vi "AMI Request Compose.vi"(7 "Checksum used":bool=TRUE, 11 "Address":u8=1) -> (3 "Request":string, 4 "Command":string="AMI")   [LabVIEW 2015, in "Samwontech TEMP2xxx.lvlib"]
uses:
  Samwontech TEMP2xxx.lvlib
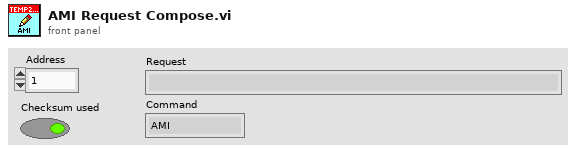
[diagram p1: front panel]
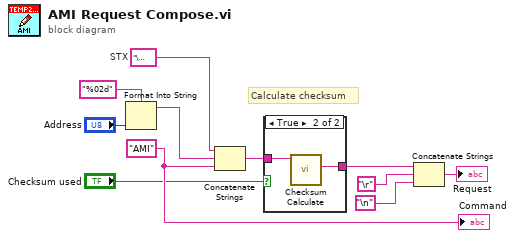
[diagram p0: block diagram]
diagram:
  w9 = "AMI" ("format string")
  w6 = "\u0002"  # STX
  # "Calculate checksum"
  n1 = Format Into String(format string="%02d", "Address") -> (resulting string=w10:string)  [unwired: 2 in, 1 out]
  n2 = Concatenate Strings(w6, w10, w9) -> (w5:string)
  n3 = case shown="True" "Checksum used" {
    tunnel: w5 -> [w12 w14]
    tunnel: [w12 w13] -> w4
    frame False {
    }
    frame True {
      n4 = call "Checksum Calculate.vi"("Command in"=w14) -> ("Command out (with checksum)"=w13:string)  [unwired: 7 in, 3 out]
    }
  }
  n5 = Concatenate Strings(w4, "\r", "\n") -> (→"Request":string)
  "Command" <- w9
